vi "Test.vi"(8 "error in (no error)":errorcluster, 11 "PreStep in":refnum<class "PreStep.lvclass">) -> (0 "error out":errorcluster, 2 "Pass?":bool, 3 "PreStep out":refnum<class "PreStep.lvclass">)   [LabVIEW 2020, in "PreStep.lvclass"]
uses:
  PreStep.lvclass
  Base Decorator/Base Decorator.lvclass
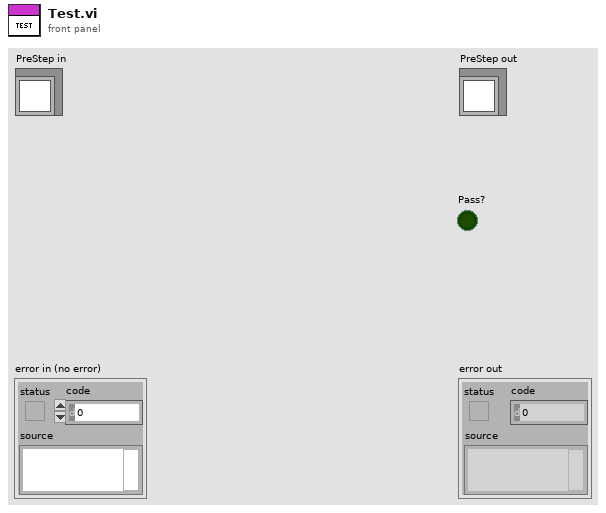
[diagram p1: front panel]
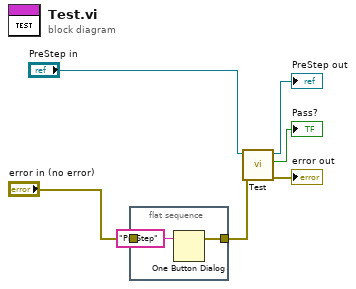
[diagram p0: block diagram]
diagram:
  n1 = flat-sequence {
    tunnel: "error in (no error)" -> [w7]
    tunnel: [w7] -> w1
    frame #0 {
      n2 = One Button Dialog(message="PreStep") -> ()  [unwired: 1 in, 1 out]
    }
  }
  n3 = call-parent "Test.vi"("error in (no error)"=w1, "Base Decorator in"="PreStep in") -> ("error out"=→"error out":errorcluster, "Pass?"=→"Pass?":bool, "Base Decorator out"=→"PreStep out":refnum<class "PreStep.lvclass">)  [unwired: 7 in]
